vi "Vsg Step SubVI.vi"(11 "file (use dialog) in":path) -> (3 "Numeric":dbl)   [LabVIEW 2016]
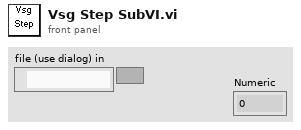
[diagram p1: front panel]
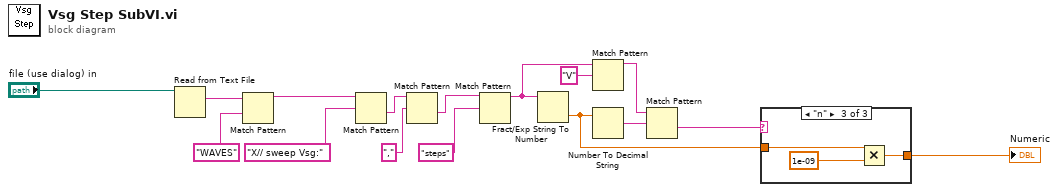
[diagram p0: block diagram]
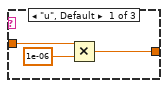
[diagram p2: hidden frame]
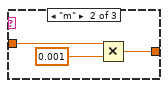
[diagram p3: hidden frame]
diagram:
  n1 = Read from Text File(file (use dialog)="file (use dialog) in") -> (text=w3:string)  [unwired: 2 in, 4 out]
  n2 = Match Pattern(string=w3, regular expression="WAVES") -> (before substring=w5:string)  [unwired: 4 out]
  n3 = Match Pattern(string=w5, regular expression="X// sweep Vsg:") -> (after substring=w7:string)  [unwired: 4 out]
  n4 = Match Pattern(string=w7, regular expression=",") -> (after substring=w9:string)  [unwired: 4 out]
  n5 = Match Pattern(string=w9, regular expression="steps") -> (before substring=w1:string)  [unwired: 4 out]
  n6 = Fract/Exp String To Number(string=w1) -> (number=w15:dbl)  [unwired: 3 in, 1 out]
  n7 = Match Pattern(string=w1, regular expression="V") -> (before substring=w13:string)  [unwired: 4 out]
  n8 = Number To Decimal String(number=w15) -> (decimal integer string=w12:string)  [unwired: 1 in]
  n9 = Match Pattern(string=w13, regular expression=w12) -> (after substring=w14:string)  [unwired: 4 out]
  n10 = case shown="\"n\"" w14 {
    tunnel: w15 -> [w18 w21 w24]
    tunnel: [w17 w20 w23] -> w16
    frame "u", Default {
      n11 = Multiply(x=w18, y=1e-06) -> (x*y=w17:dbl)
    }
    frame "m" {
      n12 = Multiply(x=w21, y=0.001) -> (x*y=w20:dbl)
    }
    frame "n" {
      n13 = Multiply(x=w24, y=1e-09) -> (x*y=w23:dbl)
    }
  }
  "Numeric" <- w16
